vi "Destroy Stage Controller.vi"(8 "error in (no error)":errorcluster, 11 "XY Stage Controller in":refnum<class "XY Stage Controller.lvclass">) -> (0 "error out":errorcluster, 3 "XY Stage Controller out":refnum<class "XY Stage Controller.lvclass">)   [LabVIEW 2022 SP3, in "XY Stage Controller.lvclass"]
uses:
  XY Stage Controller.lvclass
  Process Framework/Interlock Q Class/Interlock Q Class.lvclass
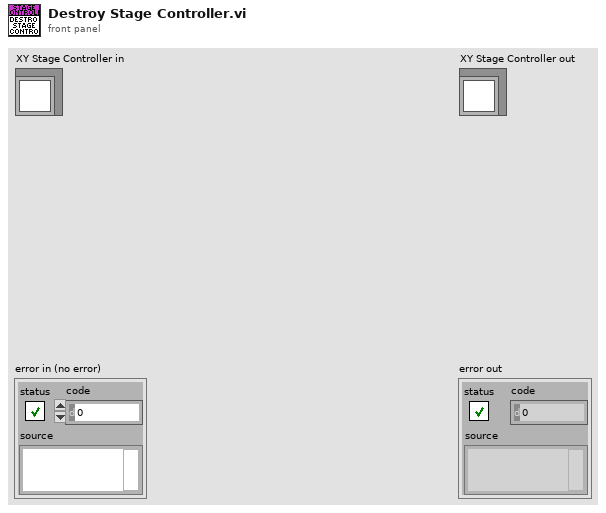
[diagram p1: front panel]
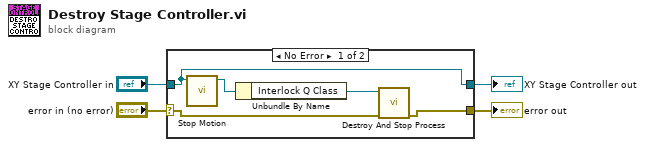
[diagram p0: block diagram]
diagram:
  n1 = case shown="No Error" "error in (no error)" {
    selector: "error in (no error)" -> [w6 w11]
    tunnel: [w5 w11] -> w3
    tunnel: [w9 w10] -> w1
    tunnel: "XY Stage Controller in" -> [w9 w10]
    frame No Error {
      n2 = call-dynamic "Stop Motion.vi"("2-Axis Stage in"=w9) -> ("2-Axis Stage out"=w8:refnum<class "XY Stage Controller.lvclass">)  [unwired: 9 in, 1 out]
      n3 = Unbundle By Name(w8) -> ("Interlock Q Class"=w7:refnum<class "Interlock Q Class.lvclass">)
      n4 = call-dynamic "Destroy And Stop Process.vi"("error in (no error)"=w6, "Interlock Q Class in"=w7) -> ("error out"=w5:errorcluster)  [unwired: 8 in, 1 out]
    }
    frame Error {
    }
  }
  "error out" <- w3
  "XY Stage Controller out" <- w1
